vi "test Deployment Import Configuration - Version 1.0.vi"(8 "error in":errorcluster, 11 "TestCase in":refnum<class "Deployment.lvclass">) -> (0 "error out":errorcluster, 3 "TestCase out":refnum<class "Deployment.lvclass">)   [LabVIEW 2020, in "Deployment.lvclass"]
uses:
  Deployment.lvclass
  Deployment.lvclass/Deployment.ctl
  315b1c3a-44c8-49e8-b756-01f865c29b4a.vi
  <vilib>/addons/_JKI Toolkits/VI Tester/TestCase.llb/TestCase.lvclass
  <vilib>/NI/VeriStand Custom Device Testing Tools/VeriStandTestUtilities/VeriStandTestUtilities.lvlib
  Scripting/Ballard MIL-STD-1553 Scripting.lvlib
  C:/Program Files (x86)/National Instruments/LabVIEW 2020/vi.lib/addons/_JKI Toolkits/VI Tester/TestCase.llb/TestCase.lvclass
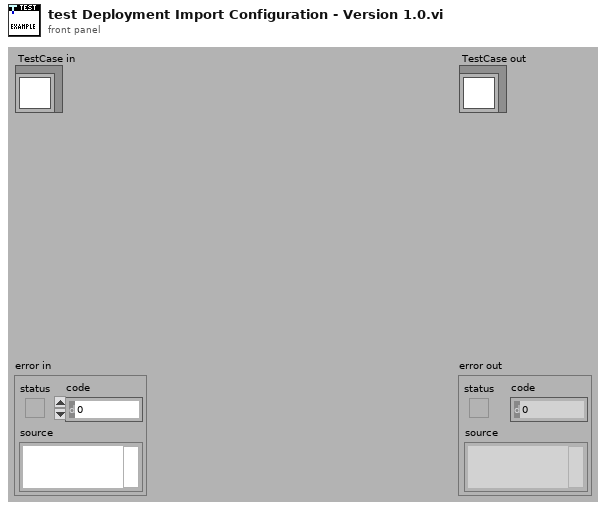
[diagram p1: front panel]
types:
  T1 = typedef "Custom Device API.lvlib/Custom Device Item Ref.ctl" = u64
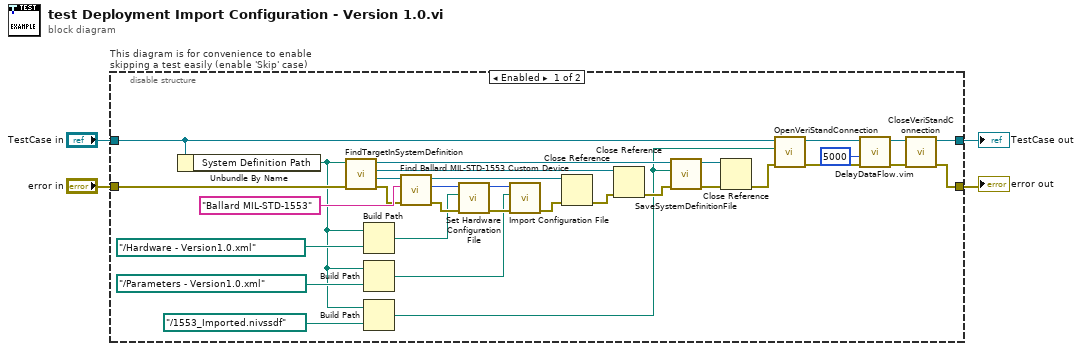
[diagram p0: block diagram]
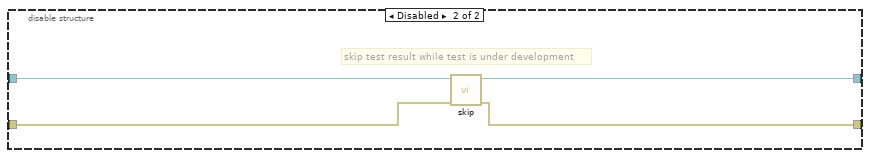
[diagram p2: hidden frame]
diagram:
  n1 = disable-structure "This diagram is for convenience to enable skipping a test easily (enable 'Skip' case)" shown="Enabled" {
    disable-tunnel: "TestCase in" -> [w29 w39]
    disable-tunnel: [w30 w37] -> w1
    disable-tunnel: [w32 w38] -> w3
    disable-tunnel: "error in" -> [w28 w36]
    frame Enabled {
      n2 = Unbundle By Name(w29) -> ("System Definition Path"=w5:path)
      n3 = call <vilib>:"FindTargetInSystemDefinition.vi"("error in"=w28, "system definition path"=w5) -> ("error out"=w16:errorcluster, "Target"=w19:refnum<k24>, "Root"=w22:refnum<k24>, "System Definition"=w27:refnum<k24>)  [unwired: 6 in]
      n4 = Build Path(base path=w5, name or relative path=path "../Hardware - Version1.0.xml" ("hardware configuration file path")) -> (appended path=w7:path)
      n5 = Build Path(base path=w5, name or relative path=path "../Parameters - Version1.0.xml" ("hardware configuration file path")) -> (appended path=w6:path)
      n6 = Build Path(base path=w5, name or relative path=path "../1553_Imported.nivssdf") -> (appended path=w13:path)
      n7 = call "Find Ballard MIL-STD-1553 Custom Device.vi"("error in"=w16, "name"="Ballard MIL-STD-1553", "target in"=w19) -> ("error out"=w14:errorcluster, "Ballard MIL-STD 1553 custom device"=w15:T1, "target out"=w17:refnum<k24>)  [unwired: 5 in, 1 out]
      n8 = call "Set Hardware Configuration File.vi"("error in"=w14, "hardware configuration file path"=w7, "Ballard MIL-STD 1553 custom device in"=w15) -> ("error out"=w12:errorcluster, "Ballard MIL-STD 1553 custom device out"=w10:T1)  [unwired: 7 in]
      n9 = call "Import Configuration File.vi"("error in"=w12, "parameters configuration file path"=w6, "Ballard MIL-STD 1553 custom device in"=w10) -> ("error out"=w11:errorcluster)  [unwired: 7 in, 1 out]
      n10 = Close Reference(reference=w17, error in (no error)=w11) -> (error out=w20:errorcluster)
      n11 = Close Reference(reference=w22, error in (no error)=w20) -> (error out=w21:errorcluster)
      n12 = call <vilib>:"SaveSystemDefinitionFile.vi"("error in (no error)"=w21, "System Definition File in"=w13, "System Definition Reference in"=w27) -> ("error out"=w24:errorcluster, "System Definition Reference out"=w25:refnum<k24>)  [unwired: 7 in]
      n13 = Close Reference(reference=w25, error in (no error)=w24) -> (error out=w23:errorcluster)
      n14 = call-dynamic "OpenVeriStandConnection.vi"("error in (no error)"=w23, "System Definition File"=w13, "VeriStand Test Case in"=w29) -> ("error out"=w35:errorcluster, "VeriStand Test Case out"=w31:refnum<class "Deployment.lvclass">)  [unwired: 6 in, 1 out]
      n15 = call "DelayDataFlow.vim"("value in"=w35, "milliseconds to wait"=u32 5000) -> ("value out"=w33:errorcluster)  [unwired: 2 in, 1 out]
      n16 = call-dynamic "CloseVeriStandConnection.vi"("error in (no error)"=w33, "VeriStand Test Case in"=w31) -> ("error out"=w32:errorcluster, "VeriStand Test Case out"=w30:refnum<class "Deployment.lvclass">)  [unwired: 8 in]
    }
    frame Disabled {
      # "skip test result while test is under development"
      n17 = call <vilib>:"skip.vi"("error in (no error)"=w36, "TestCase in"=w39) -> ("error out"=w38:errorcluster, "TestCase out"=w37:refnum<class "Deployment.lvclass">)  [unwired: 8 in]
    }
  }
  "error out" <- w3
  "TestCase out" <- w1
